vi "test_homemade_queue.vi"() -> ()   [LabVIEW 2014]
doc: "This VI performs real-time Joint-Time Frequency Analysis (JTFA) using the STFT Spectrogram PtByPt VI. The signal is simulated by a sine wave plus Gaussian noise."
uses:
  <vilib>/sound2/lvsound2.llb/Sampling Mode.ctl
  <vilib>/sound2/lvsound2.llb/Sound Data Format.ctl
  <vilib>/sound2/lvsound2.llb/Sound Input Read (DBL).vi
  <vilib>/imath/engines/lvmath2/RunTimeEngine/ArithmeticOperatorToken/NIMS_ArithmeticOperator_times.vi
  <instcachedir>/0/NIMS_ArithmeticOperator_times_831F30C6BFCCF94698B6F46369084E97.lvgen/NIMS_ArithmeticOperator_times_831F30C6BFCCF94698B6F46369084E97_001.vi
  <vilib>/imath/engines/lvmath2/RunTimeEngine/IndexRead/NIMS V(S).vi
  <instcachedir>/0/NIMS V(S)_0488751826AF41519A22953C041130DC.lvgen/NIMS V(S)_0488751826AF41519A22953C041130DC_000.vi
  <vilib>/imath/engines/lvmath2/RunTimeEngine/ErrorHandling/NIMS_Create Error From Enums.vi
  <vilib>/imath/engines/lvmath2/RunTimeEngine/NodeEndStatement/NIMS_NodeEndStatement_Output.vi
  <instcachedir>/0/NIMS_NodeEndStatement_Output_53EC0D466D134D7ABD903AC30B43404B.lvgen/NIMS_NodeEndStatement_Output_53EC0D466D134D7ABD903AC30B43404B_003.vi
  <vilib>/imath/engines/lvmath2/RunTimeEngine/ErrorHandling/NIMS_Finalize Error.vi
panel:
  out "error out":errorcluster
  in  "dft size":i32(knob)=4096 scale=32.0..512.0
  out "Now writing index...":i32
  out "x*2^n":ext
  in  "log audio device buffer samples":i32(knob)=10000 scale=2.0..16.0
  out "Sampling jitter":dbl[](graph)
  out "queue contained:":i32 format="Queue contained %.0f elements"
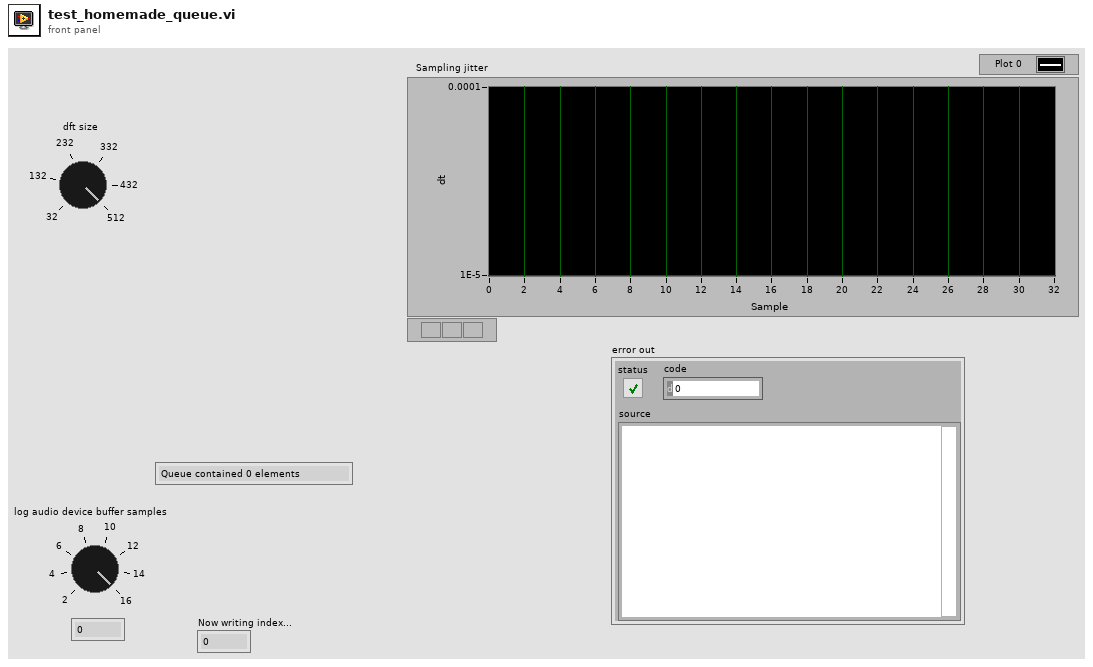
[diagram p1: front panel]
types:
  T1 = typedef "Sound Data Format.ctl" = cluster{"sample rate (S/s)":dbl, "number of channels":i32, "bits per sample":i32}
  T2 = typedef "Sampling Mode.ctl" = i32
  T3 = typedef "Sound Input Task ID.ctl" = u32
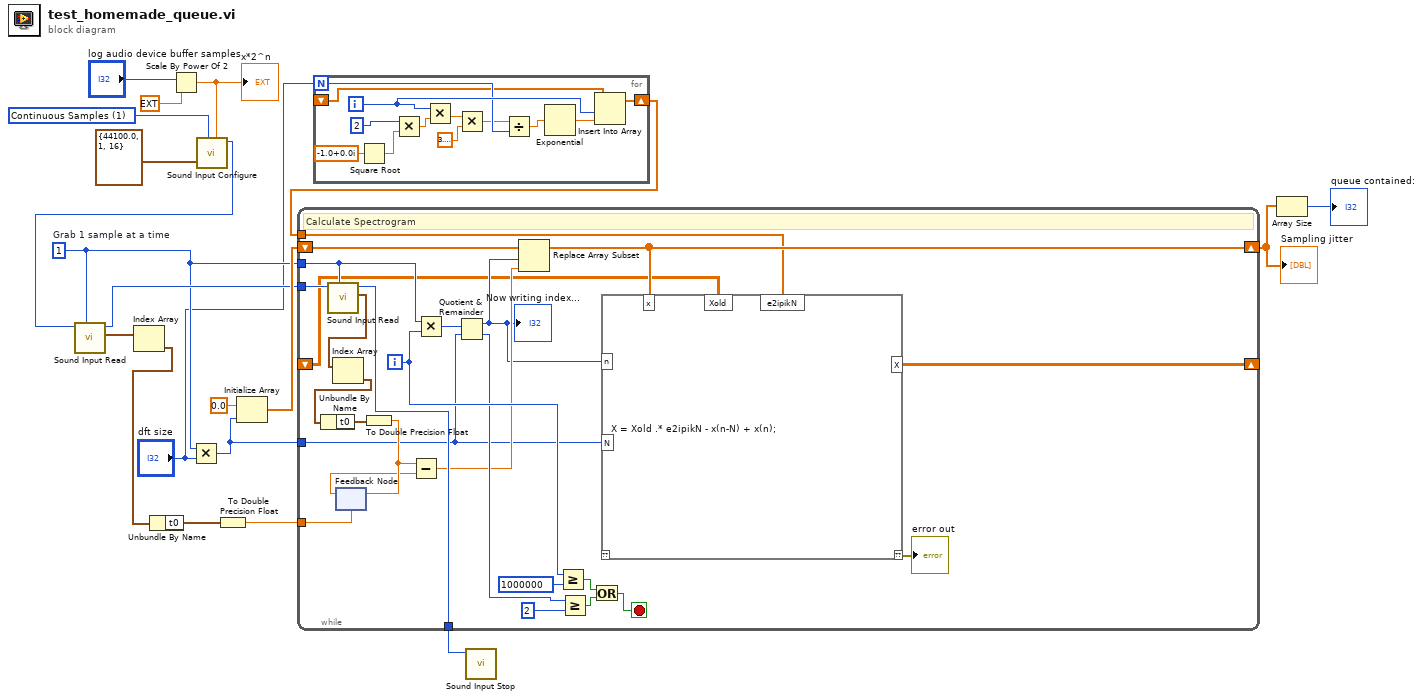
[diagram p0: block diagram]
diagram:
  w3 = 1  # Grab 1 sample at a time
  w20 = T2 1 items=["Finite Samples", "Continuous Samples"] ("sample mode")
  n1 = Scale By Power Of 2(n="log audio device buffer samples", x=ext 1.0) -> (x*2^n=w12:ext)
  "x*2^n" <- w12
  n2 = Multiply(x=w3, y="dft size") -> (x*y=w8:i32)
  n3 = call <vilib>:"Sound Input Configure.vi"("number of samples/ch"=w12, "sample mode"=w20, "sound format"=T1 {"sample rate (S/s)"=44100.0, "number of channels"=1, "bits per sample"=16}) -> ("task ID"=w18:T3)  [unwired: 7 in, 1 out]
  n4 = call-poly <vilib>:"Sound Input Read.vi"("number of samples/ch"=w3, "task ID"=w18) -> ("data"=w16:waveform(dbl)[], "task ID out"=w4:T3)  [unwired: 7 in, 1 out]
  n5 = Index Array(array=w16) -> (element=w10:waveform(dbl))  [unwired: 1 in]
  n6 = Unbundle By Name(w10) -> ("t0"=w14:timestamp)
  n7 = To Double Precision Float(number=w14) -> (double precision float=w6:dbl)
  n8 = Initialize Array(0.0 ("element"), w8) -> (w9:dbl[])
  n9 = for {
    N: "dft size" -> [w23]
    shift-right: [w33] -> w1
    shift-left: _ -> [w21]
    i -> [w27]
    n10 = Square Root(x=cdb -1.0+0.0i) -> (sqrt(x)=w30:cdb)
    n11 = Multiply(x=2, y=w30) -> (x*y=w28:cdb)
    n12 = Multiply(x=w27, y=w28) -> (x*y=w26:cdb)
    n13 = Multiply(x=w26, y=3.141592653589793) -> (x*y=w22:cdb)
    n14 = Divide(x=w22, y=w23) -> (x/y=w24:cdb)
    n15 = Exponential(1:w24) -> (0:w32:cdb)
    n16 = Insert Into Array(array=w21, index=w27, new element=w32) -> (w33:cdb[])
  }
  n17 = while {
    tunnel: w4 -> [w59]
    tunnel: w3 -> [w51]
    tunnel: [w58] -> w17
    tunnel: w6 -> [w52]
    tunnel: w8 -> [w39]
    shift-right: [w41] -> w7
    shift-left: w9 -> [w44]
    tunnel: w1 -> [w37]
    shift-right: [w36] -> _
    shift-left: _ -> [w35]
    i -> [w43]
    stop <- w47 stop-if-true
    # "Calculate Spectrogram"
    n18 = call-poly <vilib>:"Sound Input Read.vi"("number of samples/ch"=w51, "task ID"=w59) -> ("data"=w57:waveform(dbl)[], "task ID out"=w58:T3)  [unwired: 7 in, 1 out]
    n19 = Index Array(array=w57) -> (element=w56:waveform(dbl))  [unwired: 1 in]
    n20 = Unbundle By Name(w56) -> ("t0"=w55:timestamp)
    n21 = feedback #1(w52) -> (w53:dbl)
    n22 = To Double Precision Float(number=w55) -> (double precision float=w54:dbl)
    n23 = feedback-in #1(w54) -> ()
    n24 = Subtract(x=w54, y=w53) -> (x-y=w40:dbl)
    n25 = Multiply(x=w51, y=w43) -> (x*y=w50:i32)
    n26 = Quotient & Remainder(x=w50, y=w39) -> (x-y*floor(x/y)=w38:i32, floor(x/y)=w42:i32)
    "Now writing index..." <- w38
    n27 = Replace Array Subset(array=w44, new element=w40, index=w38) -> (w41:dbl[])
    n28 = Greater Or Equal?(x=w43, y=1000000) -> (x >= y?=w45:bool)
    n29 = Greater Or Equal?(x=w42, y=2) -> (x >= y?=w48:bool)
    n30 = Or(x=w45, y=w48) -> (x .or. y?=w47:bool)
    n31 = mathscript code="X = Xold .* e2ipikN - x(n-N) + x(n);"("x"=w41, "n"=w38, "N"=w39, "Xold"=w35, "e2ipikN"=w37) -> ("??"=→"error out":errorcluster, "X"=w36:cdb[][])  [unwired: 1 in]
  }
  "Sampling jitter" <- w7
  n32 = call <vilib>:"Sound Input Stop.vi"("task ID"=w17) -> ()  [unwired: 9 in, 2 out]
  n33 = Array Size(array=w7) -> (size(s)=→"queue contained:":i32)
